vi "Command & Ack - Create Endpoints.vi"(8 "error in (no error)":errorcluster, 11 "SV B-M (Host) in":refnum<class "SV B-M (Host).lvclass">) -> (0 "error out":errorcluster, 3 "SV B-M (Host) out":refnum<class "SV B-M (Host).lvclass">)   [LabVIEW 2015, in "SV B-M (Host).lvclass"]
doc: "Create command & ack network streams."
uses:
  SV B-M (Host).lvclass
  Type Defs/Message Cluster.ctl
  SV B-M (Host).lvclass/SV B-M (Host).ctl
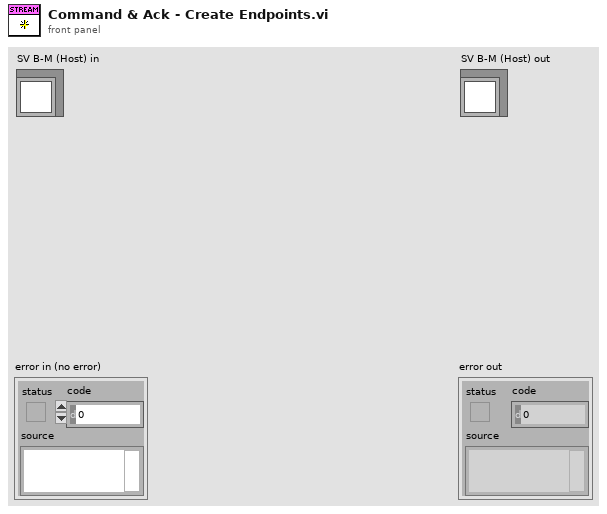
[diagram p1: front panel]
types:
  T1 = typedef "Message Cluster.ctl" = cluster{"Message":string, "Message Data":variant}
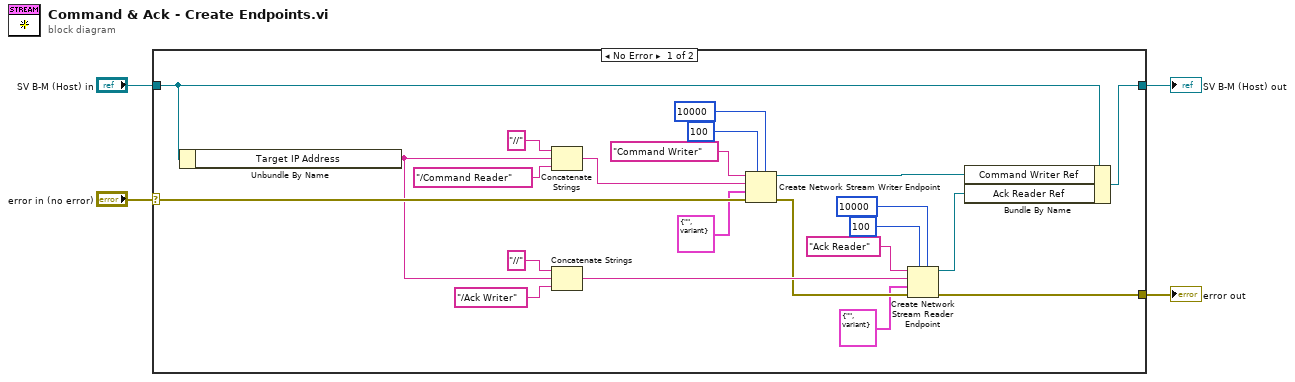
[diagram p0: block diagram]
diagram:
  n1 = case shown="No Error" "error in (no error)" {
    selector: "error in (no error)" -> [w23 w28]
    tunnel: [w9 w28] -> w3
    tunnel: [w6 w27] -> w1
    tunnel: "SV B-M (Host) in" -> [w5 w27]
    frame No Error {
      n2 = Unbundle By Name(w5) -> ("Target IP Address"=w18:string)
      n3 = Concatenate Strings("//", w18, "/Command Reader") -> (w17:string)
      n4 = Concatenate Strings("//", w18, "/Ack Writer") -> (w13:string)
      n5 = Create Network Stream Writer Endpoint(5:10000 ("timeout in ms (-1)"), 7:100 ("writer buffer size"), 8:w23, 9:T1 {"Message"="", "Message Data"=variant} ("Message Cluster"), 10:w17, 11:"Command Writer" ("writer name")) -> (0:w12:errorcluster, 3:w8:refnum<k21>)  [unwired: 1 in]
      n6 = Create Network Stream Reader Endpoint(5:10000 ("timeout in ms (-1)"), 7:100 ("writer buffer size"), 8:w12, 9:T1 {"Message"="", "Message Data"=variant} ("Message Cluster"), 10:w13, 11:"Ack Reader" ("writer name")) -> (0:w9:errorcluster, 3:w7:refnum<k21>)  [unwired: 1 in]
      n7 = Bundle By Name(cluster=w5, "Command Writer Ref"=w8, "Ack Reader Ref"=w7) -> (w6:refnum<class "SV B-M (Host).lvclass">)
    }
    frame Error {
    }
  }
  "error out" <- w3
  "SV B-M (Host) out" <- w1
